vi "Solver_002.vi"(10 "Word List":string[](array[string])=["YELLOW", "ORANGE", "PURPLE", "BLUE", "GREEN", "RED"], 11 "Word Search Grid":string[][](array[string])=[["R", "B", "L", "U", "E", "W"], ["E", "G", "N", "A", "R", "O"], ["D", "B", "C", "E", "W", "L"], ["L", "L", "D", "K", "V", "L"], ["P", "U", "R", "P", "L", "E"], ["N", "E", "E", "R", "G", "Y"]]) -> (3 "Solutions":T1={"BLUE"=[{"Row"=0, "Column"=1}, {"Row"=0, "Column"=2}, {"Row"=0, "Column"=3}, {"Row"=0, "Column"=4}], "GREEN"=[{"Row"=5, "Column"=4}, {"Row"=5, "Column"=3}, {"Row"=5, "Column"=2}, {"Row"=5, "Column"=1}, {"Row"=5, "Column"=0}], "ORANGE"=[{"Row"=1, "Column"=5}, {"Row"=1, "Column"=4}, {"Row"=1, "Column"=3}, {"Row"=1, "Column"=2}, {"Row"=1, "Column"=1}, {"Row"=1, "Column"=0}], "PURPLE"=[{"Row"=4, "Column"=0}, {"Row"=4, "Column"=1}, {"Row"=4, "Column"=2}, {"Row"=4, "Column"=3}, {"Row"=4, "Column"=4}, {"Row"=4, "Column"=5}], "RED"=[{"Row"=0, "Column"=0}, {"Row"=1, "Column"=0}, {"Row"=2, "Column"=0}], "YELLOW"=[{"Row"=5, "Column"=5}, {"Row"=4, "Column"=5}, {"Row"=3, "Column"=5}, {"Row"=2, "Column"=5}, {"Row"=1, "Column"=5}, {"Row"=0, "Column"=5}]})   [LabVIEW 2022 SP3]
uses:
  support/Solutions--map.ctl
  support/Letter Index--cluster.ctl
panel:
  # "Do not change the connector pane of this VI."
  # "Observe the default values stored in this VI to understand how each word is represented in the Solutions map.\n\nSee the block diagram for a simple implementation of a solution. Note that this approach is not very efficient, and you will want to come up with a faster way to find the words in the grid."
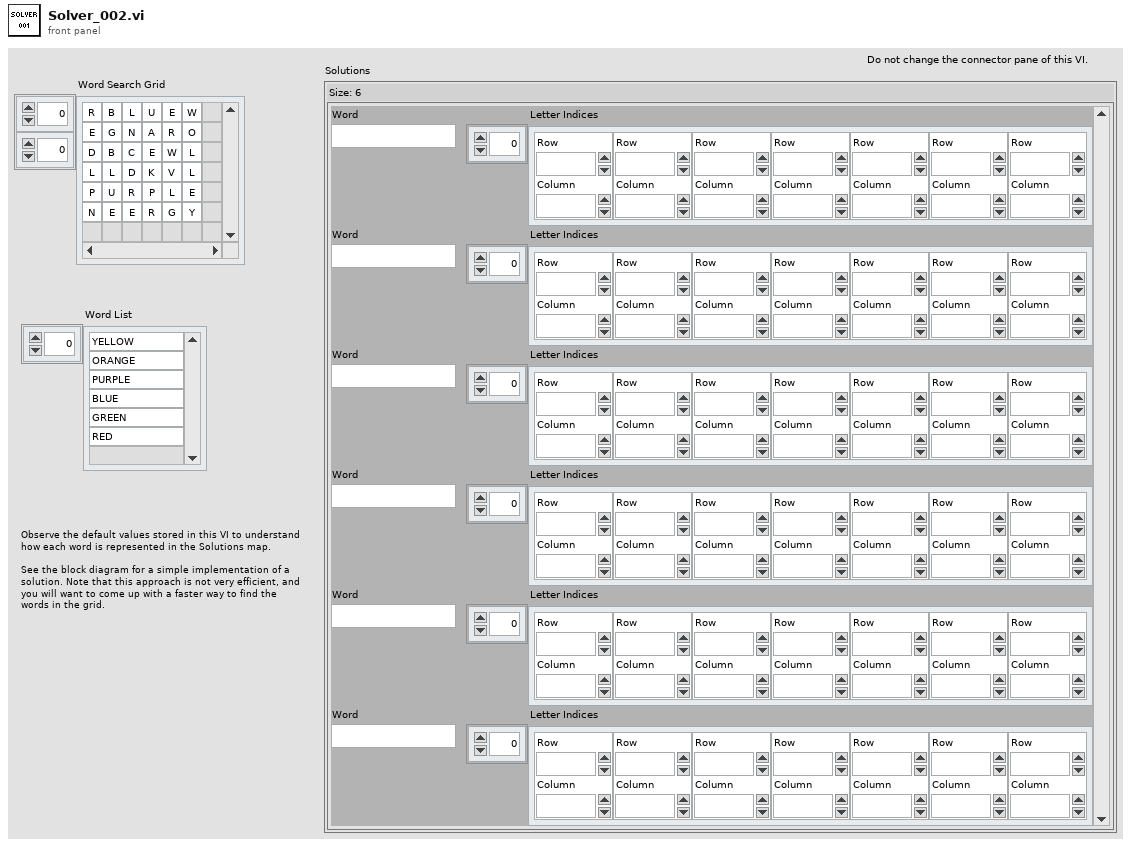
[diagram p1: front panel]
types:
  T1 = typedef "Solutions--map.ctl" = map{string, T2[]}
  T2 = typedef "Letter Index--cluster.ctl" = cluster{"Row":i32, "Column":i32}
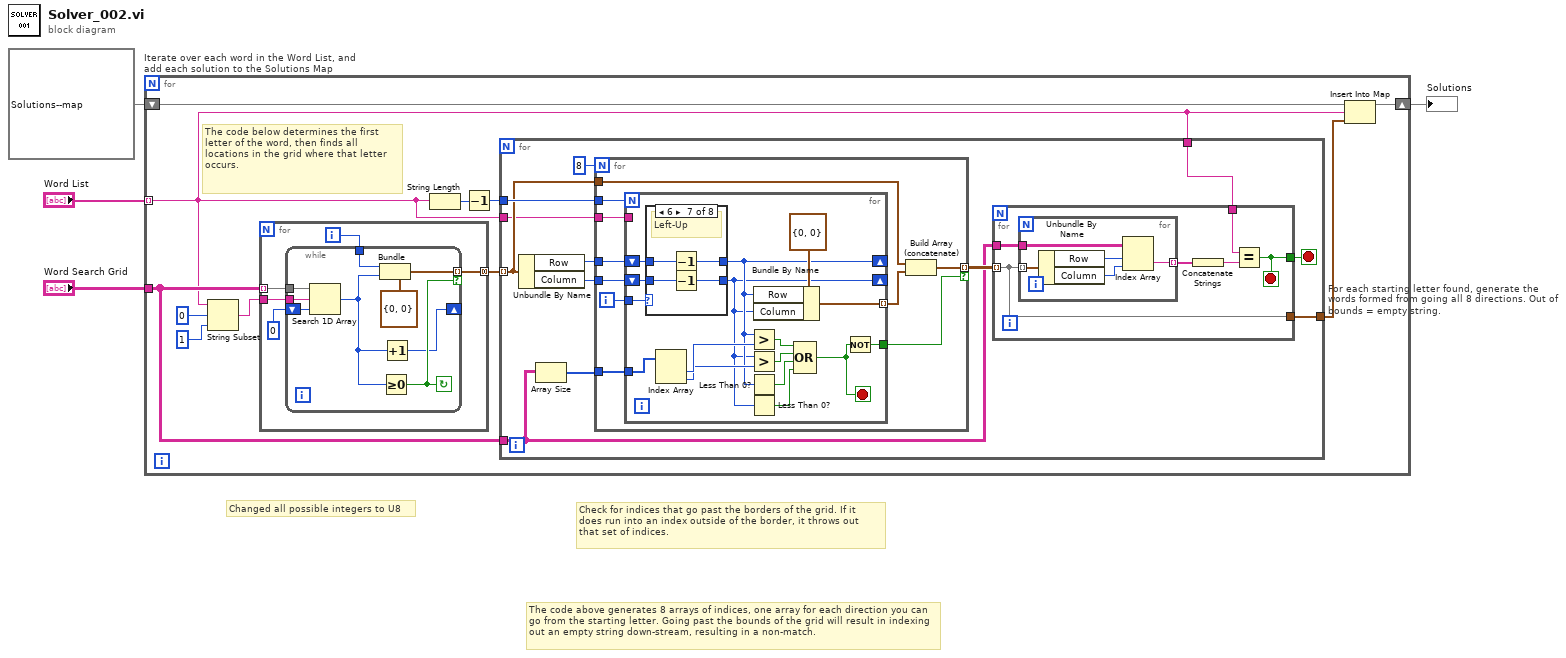
[diagram p0: block diagram]
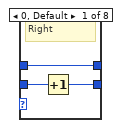
[diagram p2: hidden frame]
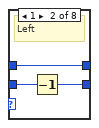
[diagram p3: hidden frame]
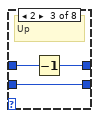
[diagram p4: hidden frame]
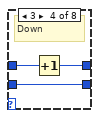
[diagram p5: hidden frame]
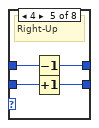
[diagram p6: hidden frame]
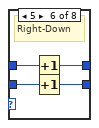
[diagram p7: hidden frame]
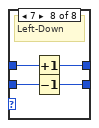
[diagram p8: hidden frame]
diagram:
  # "Check for indices that go past the borders of the grid. If it \ndoes run into an index outside of the border, it throws out\nthat set of indices."
  # "Changed all possible integers to U8"
  # "The code above generates 8 arrays of indices, one array for each direction you can go from the starting letter. Going past the bounds of the grid will result in indexing out an empty string down-stream, resulting in a non-match."
  n1 = for "Iterate over each word in the Word List, and add each solution to the Solutions Map" {
    tunnel: "Word Search Grid" -> [w7]
    tunnel: "Word List" -> [w5] mode=indexing
    shift-right: [w14] -> w4
    shift-left: T1 {} ("Solutions") -> [w15]
    # "The code below determines the first letter of the word, then finds all locations in the grid where that letter occurs."
    n2 = String Subset(string=w5, offset (0)=u8 0, length (rest)=u8 1 ("length (rest)")) -> (substring=w12:string)
    n3 = for {
      tunnel: w7 -> [w97] mode=indexing
      tunnel: w12 -> [w96]
      tunnel: [w94] -> w11 mode=concatenating
      i -> [w95]
      n4 = while {
        tunnel: w97 -> [w106]
        tunnel: w96 -> [w105]
        tunnel: w95 -> [w103]
        tunnel: [w102] -> w94 mode=indexing if=w101
        shift-right: [w98] -> _
        shift-left: 0 -> [w100]
        stop <- w101 continue-if-true
        n5 = Search 1D Array(1D array=w106, element=w105, start index (0)=w100) -> (index of element=w99:i32)
        n6 = Bundle(cluster=T2 {"Row"=0, "Column"=0} ("Letter Index"), "Row"=w103, "Column"=w99) -> (w102:T2)
        n7 = Greater Or Equal To 0?(x=w99) -> (x >= 0?=w101:bool)
        n8 = Increment(x=w99) -> (x+1=w98:i32)
      }
    }
    n9 = String Length(string=w5) -> (length=w9:i32)
    n10 = Decrement(x=w9) -> (x-1=w8:i32)
    n11 = for "For each starting letter found, generate the words formed from going all 8 directions. Out of bounds = empty string." {
      tunnel: w11 -> [w23] mode=indexing
      tunnel: w8 -> [w26]
      tunnel: w7 -> [w18]
      tunnel: [w21] -> w6
      tunnel: w5 -> [w20]
      tunnel: w5 -> [w16]
      stop <- w19 stop-if-true
      n12 = Unbundle By Name(w23) -> ("Row"=w25:i32, "Column"=w24:i32)
      n13 = Array Size(array=w18) -> (size(s)=w17:i32[])
      n14 = for {
        N: 8 -> [_]
        tunnel: w26 -> [w48]
        tunnel: w25 -> [w47]
        tunnel: w24 -> [w46]
        tunnel: w23 -> [w43]
        tunnel: [w42] -> w22 mode=indexing if=w40
        tunnel: w17 -> [w41]
        tunnel: w16 -> [w39]
        i -> [w45]
        n15 = for {
          N: w48 -> [_]
          tunnel: w45 -> [w62]
          tunnel: [w60] -> w44 mode=indexing
          shift-right: [w50] -> _
          shift-left: w47 -> [w64]
          shift-right: [w49] -> _
          shift-left: w46 -> [w63]
          tunnel: w41 -> [w59]
          tunnel: [w53] -> w40
          tunnel: w39 -> [_]
          stop <- w54 stop-if-true
          n16 = case shown="6" w62 {
            tunnel: w64 -> [w65 w68 w72 w75 w79 w83 w87 w91]
            tunnel: w63 -> [w67 w70 w73 w76 w80 w84 w88 w92]
            tunnel: [w66 w69 w73 w76 w77 w81 w85 w89] -> w49
            tunnel: [w65 w68 w71 w74 w78 w82 w86 w90] -> w50
            frame 0, Default {
              # "Right"
              n17 = Increment(x=w67) -> (x+1=w66:i32)
            }
            frame 1 {
              # "Left"
              n18 = Decrement(x=w70) -> (x-1=w69:i32)
            }
            frame 2 {
              # "Up"
              n19 = Decrement(x=w72) -> (x-1=w71:i32)
            }
            frame 3 {
              # "Down"
              n20 = Increment(x=w75) -> (x+1=w74:i32)
            }
            frame 4 {
              # "Right-Up"
              n21 = Decrement(x=w79) -> (x-1=w78:i32)
              n22 = Increment(x=w80) -> (x+1=w77:i32)
            }
            frame 5 {
              # "Right-Down"
              n23 = Increment(x=w83) -> (x+1=w82:i32)
              n24 = Increment(x=w84) -> (x+1=w81:i32)
            }
            frame 6 {
              # "Left-Up"
              n25 = Decrement(x=w87) -> (x-1=w86:i32)
              n26 = Decrement(x=w88) -> (x-1=w85:i32)
            }
            frame 7 {
              # "Left-Down"
              n27 = Increment(x=w91) -> (x+1=w90:i32)
              n28 = Decrement(x=w92) -> (x-1=w89:i32)
            }
          }
          n29 = Index Array(array=w59) -> (element #1=w58:i32, element #2=w57:i32)  [unwired: 2 in]
          n30 = Greater?(x=w50, y=w58) -> (0:w56:bool)
          n31 = Greater?(x=w49, y=w57) -> (0:w55:bool)
          n32 = Less Than 0?(x=w50) -> (x < 0?=w52:bool)
          n33 = Less Than 0?(x=w49) -> (x < 0?=w51:bool)
          n34 = Bundle By Name(cluster=T2 {"Row"=0, "Column"=0} ("Letter Index"), "Row"=w50, "Column"=w49) -> (w60:T2)
          n35 = Compound Arithmetic op=OR(w56, w55, w52, w51) -> (w54:bool)
          n36 = Not(x=w54) -> (.not. x?=w53:bool)
        }
        n37 = Build Array (concatenate)(w43, w44) -> (w42:T2[])
      }
      n38 = for {
        tunnel: w22 -> [w30] mode=indexing
        tunnel: w18 -> [w33]
        tunnel: [w30] -> w21
        tunnel: w20 -> [w29]
        tunnel: [w28] -> w19
        stop <- w28 stop-if-true
        n39 = for {
          tunnel: w30 -> [w38] mode=indexing
          tunnel: w33 -> [w36]
          tunnel: [w34] -> w32 mode=indexing
          n40 = Unbundle By Name(w38) -> ("Row"=w37:i32, "Column"=w35:i32)
          n41 = Index Array(array=w36, index (row)=w37, index (col)=w35) -> (element=w34:string)
        }
        n42 = Concatenate Strings(w32) -> (w31:string)
        n43 = Equal?(x=w29, y=w31) -> (x = y?=w28:bool)
      }
    }
    n44 = Insert Into Map(map in=w15, key=w5, value=w6) -> (map out=w14:T1)  [unwired: 2 out]
  }
  "Solutions" <- w4
